vi "Get DAQmxTask.vi"(8 "error in (no error)":errorcluster, 10 "Task name":string, 11 "DAQmxTaskContainer in":refnum<class "DAQmxTaskContainer.lvclass">) -> (0 "error out":errorcluster, 2 "DAQmx Task":refnum<class "DAQmxTask.lvclass">, 3 "DAQmxTaskContainer out":refnum<class "DAQmxTaskContainer.lvclass">)   [LabVIEW 2015, in "DAQmxTaskContainer.lvclass"]
uses:
  DAQmxTaskContainer.lvclass
  DAQmxTask.lvclass
  DAQmxTaskContainer.lvclass/DAQmxTaskContainer.ctl
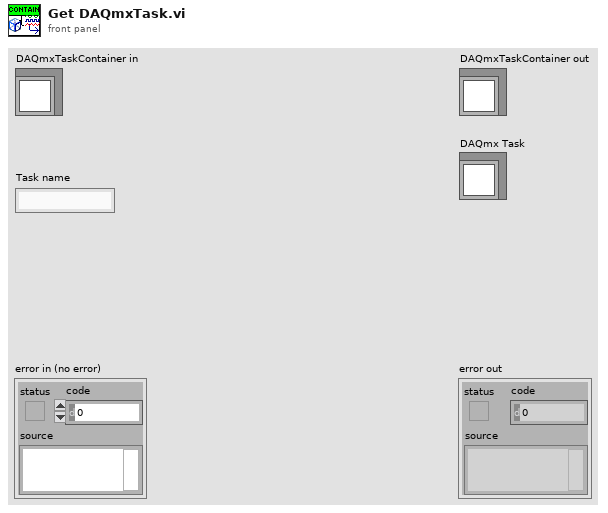
[diagram p1: front panel]
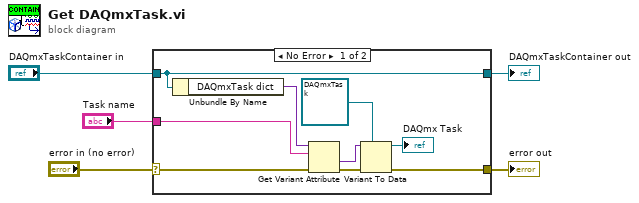
[diagram p0: block diagram]
diagram:
  n1 = case shown="No Error" "error in (no error)" {
    selector: "error in (no error)" -> [w11 w16]
    tunnel: [w8 w16] -> w4
    tunnel: [w14 w15] -> w2
    tunnel: "DAQmxTaskContainer in" -> [w14 w15]
    tunnel: "Task name" -> [w12 _]
    frame No Error {
      n2 = Unbundle By Name(w14) -> ("DAQmxTask dict"=w13:variant)
      n3 = Get Variant Attribute(Variant=w13, name=w12, error in=w11) -> (value=w10:variant, error out=w9:errorcluster)  [unwired: 1 in, 2 out]
      n4 = Variant To Data(error in=w9, type=refnum<class "DAQmxTask.lvclass"> refnum ("DAQmxTask.lvclass"), Variant=w10) -> (data=→"DAQmx Task":refnum<class "DAQmxTask.lvclass">, error out=w8:errorcluster)
    }
    frame Error {
    }
  }
  "error out" <- w4
  "DAQmxTaskContainer out" <- w2
